vi "Drive PID Controller.vi"(4 "reinitialize? (F)":bool, 5 "Turn Only?":bool, 6 "High Gear?":bool, 7 "Speed Limits":T3={"Turn Speed Limits"={"upper limit"=1.0, "lower limit"=1.0}, "Straight Speed Limits"={"upper limit"=1.0, "lower limit"=1.0}}, 8 "From Shift":T1, 9 "Procces Variable":cluster{"Angle":dbl, "Encoder Distance":dbl}, 10 "Setpoints":T5, 11 "PID Gains":T4) -> (0 "To Shift":T2, 2 "Throttle output":dbl, 3 "Steer ouput":dbl)   [LabVIEW 2013]
uses:
  <vilib>/addons/control/pid/pid.llb/PID (DBL).vi
  <vilib>/addons/control/pid/NI_PID_pid.lvlib
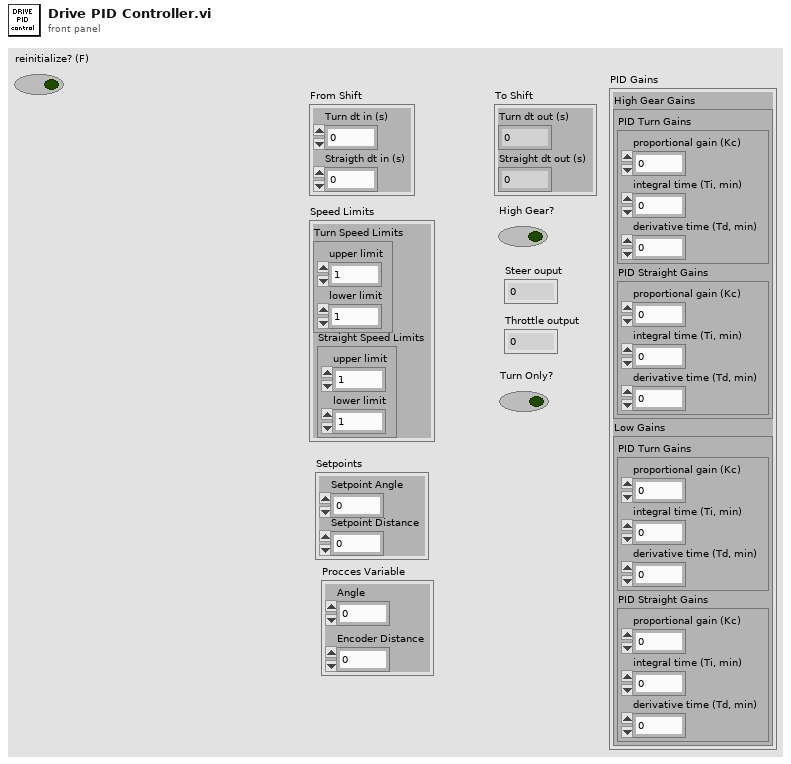
[diagram p1: front panel]
types:
  T1 = cluster{"Turn dt in (s)":dbl, "Straigth dt in (s)":dbl}
  T2 = cluster{"Turn dt out (s)":dbl, "Straight dt out (s)":dbl}
  T3 = cluster{"Turn Speed Limits":cluster{"upper limit":dbl, "lower limit":dbl}, "Straight Speed Limits":cluster{"upper limit":dbl, "lower limit":dbl}}
  T4 = cluster{"High Gear Gains":cluster{"PID Turn Gains":cluster{"proportional gain (Kc)":dbl, "integral time (Ti, min)":dbl, "derivative time (Td, min)":dbl}, "PID Straight Gains":cluster{"proportional gain (Kc)":dbl, "integral time (Ti, min)":dbl, "derivative time (Td, min)":dbl}}, "Low Gains":cluster{"PID Turn Gains":cluster{"proportional gain (Kc)":dbl, "integral time (Ti, min)":dbl, "derivative time (Td, min)":dbl}, "PID Straight Gains":cluster{"proportional gain (Kc)":dbl, "integral time (Ti, min)":dbl, "derivative time (Td, min)":dbl}}}
  T5 = cluster{"Setpoint Angle":dbl, "Setpoint Distance":dbl}
  T6 = cluster{"PID Turn Gains":cluster{"proportional gain (Kc)":dbl, "integral time (Ti, min)":dbl, "derivative time (Td, min)":dbl}, "PID Straight Gains":cluster{"proportional gain (Kc)":dbl, "integral time (Ti, min)":dbl, "derivative time (Td, min)":dbl}}
  T7 = cluster{"proportional gain (Kc)":dbl, "integral time (Ti, min)":dbl, "derivative time (Td, min)":dbl}
  T8 = cluster{"dt out (s)":dbl, "Encoder Distance":dbl}
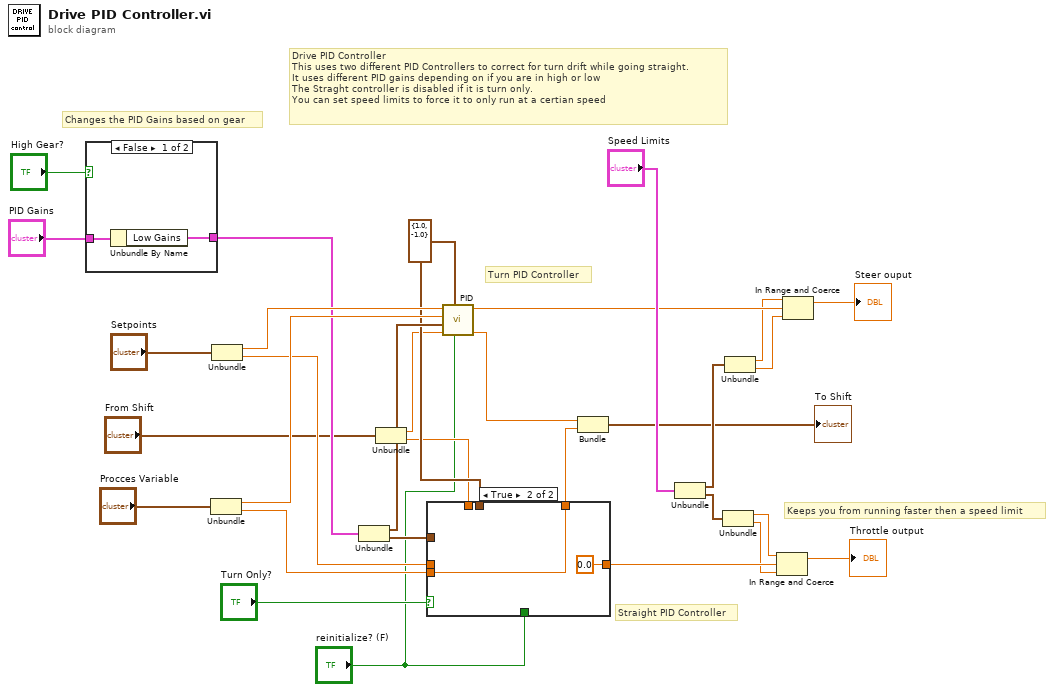
[diagram p0: block diagram]
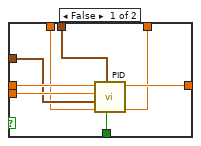
[diagram p2: hidden frame]
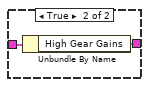
[diagram p3: hidden frame]
diagram:
  w20 = cluster{"output high":dbl, "output low":dbl} {"output high"=1.0, "output low"=-1.0} ("output range")
  # "Changes the PID Gains based on gear"
  # "Keeps you from running faster then a speed limit"
  # "Straight PID Controller"
  # "Turn PID Controller"
  # "Drive PID Controller\nThis uses two different PID Controllers to correct for turn drift while going straight.\nIt uses different PID gains depending on if you are in high or low\nThe Straght controller is disabled if it is turn only.\nYou can set speed limits to force it to only run at a certian speed"
  n1 = case shown="False" "High Gear?" {
    tunnel: "PID Gains" -> [w33 w35]
    tunnel: [w32 w34] -> w23
    frame False {
      n2 = Unbundle By Name(w33) -> ("Low Gains"=w32:T6)
    }
    frame True {
      n3 = Unbundle By Name(w35) -> ("High Gear Gains"=w34:T6)
    }
  }
  n4 = Unbundle("Procces Variable") -> ("Angle"=w28:dbl, "Encoder Distance"=w26:dbl)
  n5 = Unbundle("Setpoints") -> ("Setpoint Angle"=w30:dbl, "Setpoint Distance"=w27:dbl)
  n6 = Unbundle(w23) -> ("PID Turn Gains"=w22:T7, "PID Straight Gains"=w21:T7)
  n7 = Unbundle("From Shift") -> ("Turn dt in (s)"=w6:dbl, "Straigth dt in (s)"=w5:dbl)
  n8 = case shown="True" "Turn Only?" {
    tunnel: w27 -> [w43 _]
    tunnel: w26 -> [w42 w45]
    tunnel: w21 -> [w41 _]
    tunnel: w20 -> [w40 _]
    tunnel: [w39 0.0 ("output")] -> w13
    tunnel: [w38 w45] -> w9
    tunnel: w5 -> [w37 _]
    tunnel: "reinitialize? (F)" -> [w36 _]
    frame False {
      n9 = call-poly <vilib>:"PID.vi"("reinitialize? (F)"=w36, "output range"=w40, "dt (s)"=w37, "PID gains"=w41, "process variable"=w42, "setpoint"=w43) -> ("dt out (s)"=w38:dbl, "output"=w39:dbl)  [unwired: 4 in]
    }
    frame True {
    }
  }
  n10 = call-poly <vilib>:"PID.vi"("reinitialize? (F)"="reinitialize? (F)", "output range"=w20, "dt (s)"=w6, "PID gains"=w22, "process variable"=w28, "setpoint"=w30) -> ("dt out (s)"=w10:dbl, "output"=w18:dbl)  [unwired: 4 in]
  n11 = Bundle("dt out (s)"=w10, "Encoder Distance"=w9) -> (→"To Shift":T8)  [unwired: 1 in]
  n12 = Unbundle("Speed Limits") -> ("Turn Speed Limits"=w17:cluster{"upper limit":dbl, "lower limit":dbl}, "Straight Speed Limits"=w14:cluster{"upper limit":dbl, "lower limit":dbl})
  n13 = Unbundle(w14) -> ("upper limit"=w11:dbl, "lower limit"=w12:dbl)
  n14 = Unbundle(w17) -> ("upper limit"=w16:dbl, "lower limit"=w15:dbl)
  n15 = In Range and Coerce(upper limit=w11, x=w13, lower limit=w12) -> (coerced(x)=→"Throttle output":dbl)  [unwired: 1 out]
  n16 = In Range and Coerce(upper limit=w16, x=w18, lower limit=w15) -> (coerced(x)=→"Steer ouput":dbl)  [unwired: 1 out]
